vi "Read Current Actual.vi"   [LabVIEW 2023, in "Cycler.lvclass"]
uses:
  Cycler.lvclass
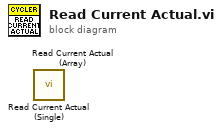
[diagram p0: block diagram]
diagram:
  n1 = call "Read Current Actual (Single).vi"() -> ()  [unwired: 8 in, 4 out]
  n2 = call "Read Current Actual (Array).vi"() -> ()  [unwired: 8 in, 4 out]
